vi "Supported Smart Syntax Representation.vi"(0 "Bitwise Operations in":refnum<class "Bitwise Functions.lvclass">, 11 "error in (no error)":errorcluster) -> (4 "Bitwise Operations out":refnum<class "Bitwise Functions.lvclass">, 6 "Smart Syntax Representation List":string[](array[string]), 15 "error out":errorcluster)   [LabVIEW 2019, in "Bitwise Functions.lvclass"]
uses:
  Bitwise Functions.lvclass
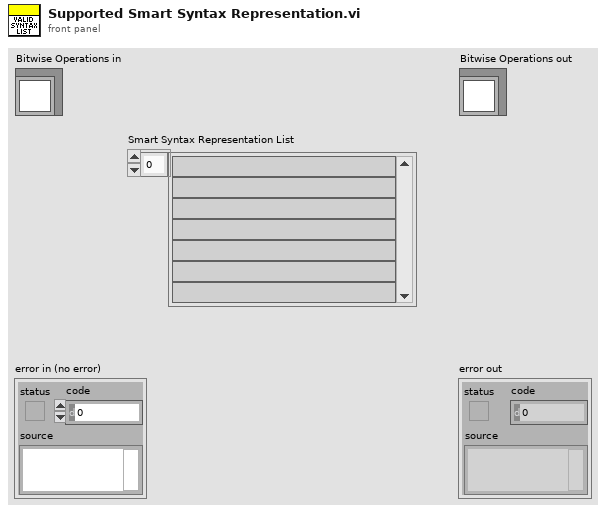
[diagram p1: front panel]
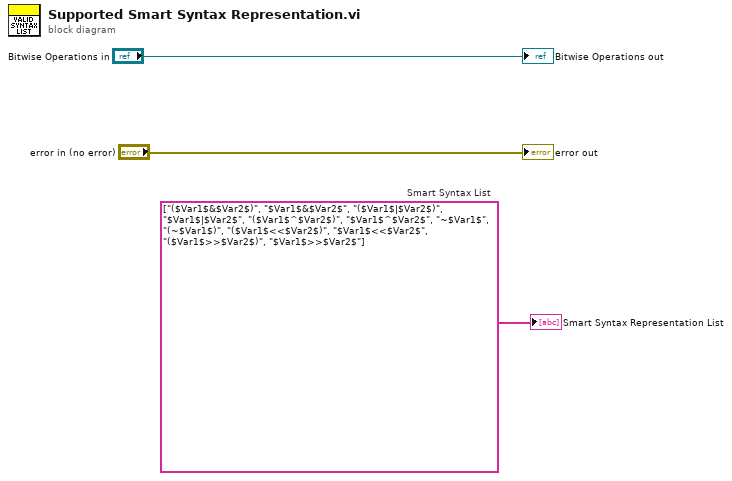
[diagram p0: block diagram]
diagram:
  w1 = string[] ["($Var1$&$Var2$)", "$Var1$&$Var2$", "($Var1$|$Var2$)", "$Var1$|$Var2$", "($Var1$^$Var2$)", "$Var1$^$Var2$", "~$Var1$", "(~$Var1$)", "($Var1$<<$Var2$)", "$Var1$<<$Var2$", "($Var1$>>$Var2$)", "$Var1$>>$Var2$"]  # Smart Syntax List
  "error out" <- "error in (no error)"
  "Bitwise Operations out" <- "Bitwise Operations in"
  "Smart Syntax Representation List" <- w1
